vi "Open_Connection.vi"(8 "error in (no error)":errorcluster) -> (0 "error out":errorcluster, 3 "client handle out":T1)   [LabVIEW 2018, in "MerriamWebsterJSON.lvlib"]
uses:
  MerriamWebsterJSON.lvlib
  <vilib>/httpClient/ClientHandle.ctl
  <vilib>/httpClient/LabVIEWHTTPClient.lvlib
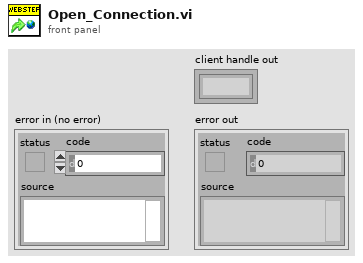
[diagram p1: front panel]
types:
  T1 = typedef "LabVIEWHTTPClient.lvlib/ClientHandle.ctl" = refnum<k1>
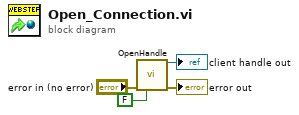
[diagram p0: block diagram]
diagram:
  n1 = call <vilib>:"OpenHandle.vi"("error in (no error)"="error in (no error)", "verify server(true)"=FALSE) -> ("client handle out"=→"client handle out":T1, "error out"=→"error out":errorcluster)  [unwired: 12 in]
